vi "Heart Rate Monitor.vi"() -> ()   [LabVIEW 2018, in "Heart Rate Monitor.lvlib"]
uses:
  Heart Rate Monitor.lvlib
  Program Files (x86)/National Instruments/LabVIEW 2018/examples/Instrument IO/Serial/support/Serial - Settings.ctl
  Program Files (x86)/National Instruments/LabVIEW 2018/examples/Instrument IO/Serial/support/Serial - XON-XOFF Characters.ctl
  Program Files (x86)/National Instruments/LabVIEW 2018/examples/Instrument IO/Serial/support/Serial - ASCII Characters.ctl
  <vilib>/Instr/_visa.llb/VISA Configure Serial Port (Instr).vi
panel:
  in  "Termination Character":u8=10 format="%.0x"
  in  "End Read on Termination Character?":bool=TRUE
  in  "Stop":bool
  out "Response":string
  in  "XON/XOFF Characters":T1={"XON"=enum."DC1", "XOFF"=enum."DC3"}
  in  "Serial Settings":T3={"baud rate"=9600, "data bits"=8, "parity"=enum."None", "stop bits"=10, "flow control"=0} {"flow control" items=["None"=0, "XON/XOFF"=1, "RTS/CTS"=2, "DTR/DSR"=4]; "stop bits" items=["1.0"=10, "1.5"=15, "2.0"=20]; "data bits" min=5 max=8 step=1; "baud rate" items=["75"=75, "110"=110, "134"=134, "150"=150, "300"=300, "600"=600, "1200"=1200, "1800"=1800, "2400"=2400, "4800"=4800, "7200"=7200, "9600"=9600, "14400"=14400, "19200"=19200, "28800"=28800, "38400"=38400, "56000"=56000, "57600"=57600, "115200"=115200, "128000"=128000, "230400"=230400]}
  in  "VISA resource name":refnum<visa-resource-name>="COM1"
  # "Overview: Demonstrates the use of the VISA functions to write commands to and read responses from a serial instrument continuously in a loop.\nRequirements: NI-VISA Driver\nInstructions:\n1. Run the VI.\n2. Specify a Command and click the Write button.\n3. Read a Response by clicking the Read button.\n4. Click Stop to stop the VI."
  # "0xA is equivalent to a '\\n' character, which is a line feed."
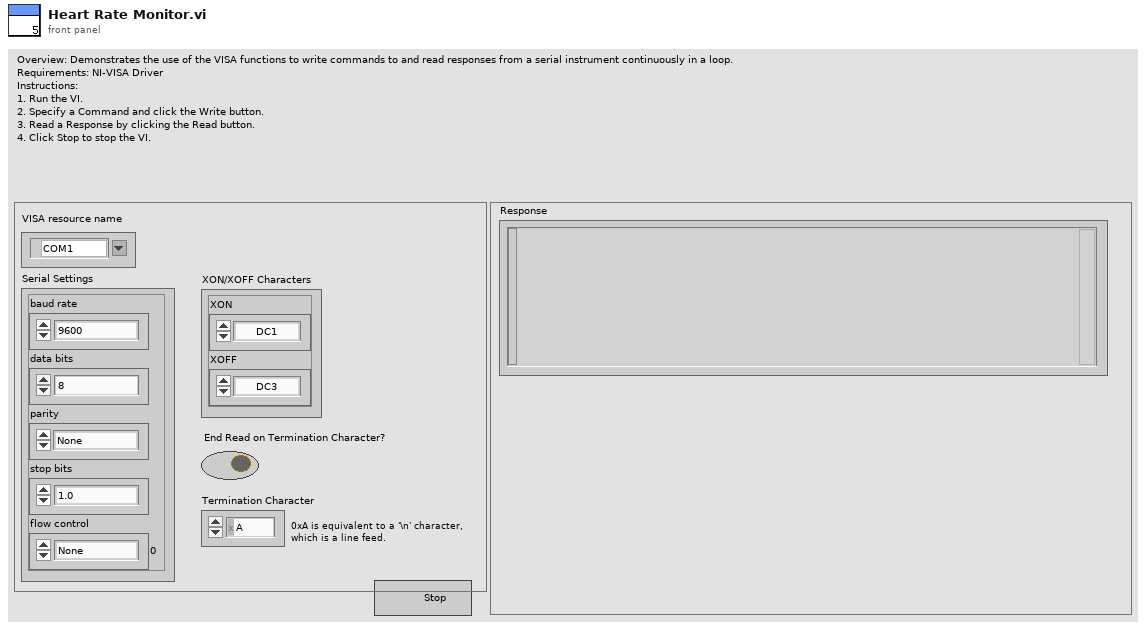
[diagram p1: front panel]
types:
  T1 = typedef "Serial - XON-XOFF Characters.ctl" = cluster{"XON":T2, "XOFF":T2}
  T2 = typedef "Serial - ASCII Characters.ctl" = enum16{"NUL", "SOH", "STX", "ETX", "EOT", "ENQ", "ACK", "BEL", "BS", "HT", "LF", "VT", "FF", "CR", "SO", "SI", "DLE", "DC1", "DC2", "DC3", "DC4", "NAK", "SYN", "ETB", "CAN", "EM", "SUB", "ESC", "FS", "GS", "RS", "US", "SP", "!", "\"", "#", "$", "%", "&", "'", "(", ")", "*", "+", ",", "- (-)", ".", "/", "0", "1", "2", "3", "4", "5", "6", "7", "8", "9", ":", ";", "<", "=", ">", "?", "@", "A", "B", "C", "D", "E", "F", "G", "H", "I", "J", "K", "L", "M", "N", "O", "P", "Q", "R", "S", "T", "U", "V", "W", "X", "Y", "Z", "[", "\\", "]", "^", "_", "`", "a", "b", "c", "d", "e", "f", "g", "h", "i", "j", "k", "l", "m", "n", "o", "p", "q", "r", "s", "t", "u", "v", "w", "x", "y", "z", "{", "|", "}", "~"}
  T3 = typedef "Serial - Settings.ctl" = cluster{"baud rate":u32, "data bits":u16, "parity":enum16{"None", "Odd", "Even", "Mark", "Space"}, "stop bits":u16, "flow control":u16}
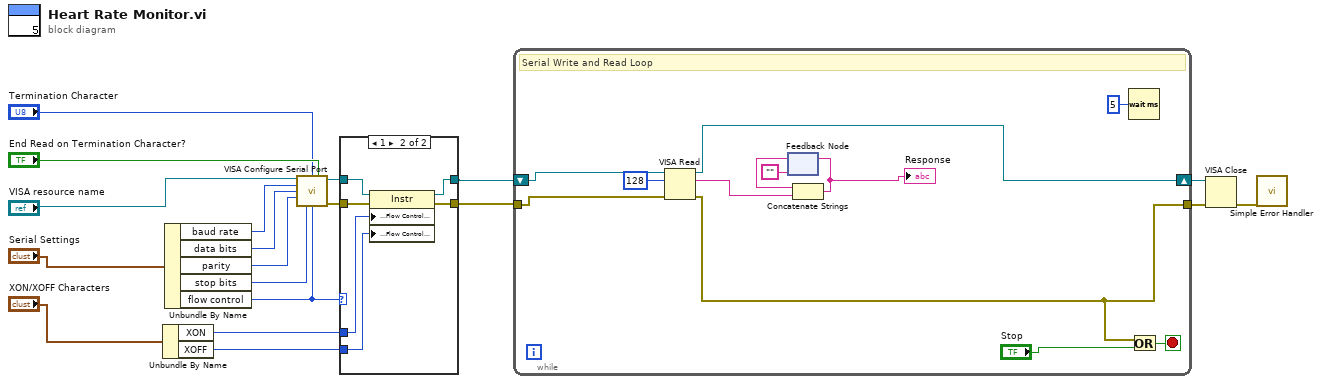
[diagram p0: block diagram]
diagram:
  n1 = Unbundle By Name("XON/XOFF Characters") -> ("XON"=w12:T2, "XOFF"=w11:T2)
  n2 = Unbundle By Name("Serial Settings") -> ("baud rate"=w14:u32, "data bits"=w15:u16, "parity"=w16:enum16{"None", "Odd", "Even", "Mark", "Space"}, "stop bits"=w17:u16, "flow control"=w13:u16)
  n3 = call-poly "VISA Configure Serial Port"("VISA resource name"="VISA resource name", "termination char\n(0xA = '\\n' = LF)"="Termination Character", "Enable Termination\nChar (T)"="End Read on Termination Character?", "baud rate (9600)"=w14, "data bits (8)"=w15, "parity (0:none)"=w16, "stop bits (10: 1 bit)"=w17, "flow control (0:none)"=w13) -> ("VISA resource name out"=w18:refnum<visa-resource-name>, "error out"=w19:errorcluster)  [unwired: 2 in, 4 out]
  n4 = case shown="1" w13 {
    tunnel: [w20 w27] -> w3
    tunnel: [w21 w26] -> w2
    tunnel: w19 -> [w20 w25]
    tunnel: w18 -> [w21 w24]
    tunnel: w12 -> [_ w23]
    tunnel: w11 -> [_ w22]
    frame Default {
    }
    frame 1 {
      n5 = property class="Instr"(reference=w24, error in=w25, "Serial Settings:Flow Control XON Character"=w23, "Serial Settings:Flow Control XOFF Character"=w22) -> (reference out=w26:refnum<visa-resource-name>, error out=w27:errorcluster)
    }
  }
  n6 = while {
    shift-right: [w34] -> w4
    shift-left: w2 -> [w29]
    tunnel: w3 -> [w32]
    tunnel: [w30] -> w5
    stop <- w38 stop-if-true
    # "Serial Write and Read Loop"
    n7 = VISA Read(VISA resource name=w29, byte count=u32 128, error in (no error)=w32) -> (VISA resource name out=w34:refnum<visa-resource-name>, read buffer=w35:string, error out=w30:errorcluster)  [unwired: 1 out]
    n8 = feedback #1("") -> (w37:string)
    n9 = Concatenate Strings(w37, w35) -> (w33:string)
    "Response" <- w33
    n10 = feedback-in #1(w33) -> ()
    n11 = Wait (ms)(milliseconds to wait=u32 5) -> ()  [unwired: 1 out]
    n12 = Or(x=w30, y="Stop") -> (x .or. y?=w38:bool)
  }
  n13 = VISA Close(VISA resource name=w4, error in (no error)=w5) -> (error out=w1:errorcluster)
  n14 = call <vilib>:"Simple Error Handler.vi"("error in (no error)"=w1) -> ()  [unwired: 1 in, 8 out]
